vi "PosStrikerFollowAttacker.vi"(4 "Pos Attacker":dbl[](array[numeric]), 6 "atacando ao contrário?":bool=TRUE, 8 "IA Input":T1={"our_robots"=[], "enemy_robots"=[], "balls"=[], "geometry"={"line_width"=0, "field_length"=0, "field_width"=0, "boundary_width"=0, "referee_width"=0, "goal_width"=0, "goal_depth"=0, "goal_wall_width"=0, "center_circle_radius"=0, "defense_radius"=0, "defense_stretch"=0, "free_kick_from_defense_dist"=0, "penalty_spot_from_field_line_dist"=0, "penalty_line_from_spot_dist"=0}, "IA Judge"={"stage"="", "command"="", "our_goalie_id"=0.0, "enemy_goalie_id"=0.0, "command enum"=enum."Halt", "Time"=enum."Azul"}, "Received Timestamp"=timestamp(0 s since 1904-01-01), "Events"={"Touch"=FALSE, "Ball out"=FALSE, "id touch"=0.0, "Ball out of \nVision"=FALSE, "Ball inside \nGoalie area"=FALSE, "Robot not responding"=FALSE, "Robots responding status"=[1.0, 1.0, 1.0, 1.0, 1.0, 1.0], "Enemy Ball \nPossession"=FALSE, "Pass State"=FALSE, "id end of pass"=0.0, "Kick"=FALSE}}, 9 "balls":T5[](array[typedef])=[{"x"=-2165.869384765625, "y"=510.4085693359375, "timestamp"=timestamp(2082758857.4639893 s since 1904-01-01), "Vel_x"=0.0, "Vel_y"=0.0}], 10 "Field Size in":T6={"line_width"=10, "field_length"=6000, "field_width"=4000, "boundary_width"=250, "referee_width"=425, "goal_width"=700, "goal_depth"=180, "goal_wall_width"=20, "center_circle_radius"=500, "defense_radius"=500, "defense_stretch"=350, "free_kick_from_defense_dist"=700, "penalty_spot_from_field_line_dist"=450, "penalty_line_from_spot_dist"=350}, 11 "Robot in":T2={"id"=5, "function"=enum."Attacker", "x"=-1842.5054931640625, "y"=520.60986328125, "orientation"=-2.7555055618286133, "v_tangent"=0.0, "v_normal"=0.0, "v_ang"=0.0, "kick_x"=0.0, "kick_z"=0.0, "dribble"=FALSE, "Timestamp"=timestamp(2082758857.4639893 s since 1904-01-01), "dest_x"=0.0, "dest_y"=0.0, "dest_orientation"=0.0, "estimatives"={"est_v_tangent"=0.0, "est_v_normal"=0.0, "est_vx"=0.0, "est_vy"=0.0}, "dest_x_kick"=0.0, "dest_y_kick"=0.0, "Gap Coord"=[], "States"=enum."GoToTangent"}) -> (2 "Robot out":T2={"id"=5, "function"=enum."Attacker", "x"=-1842.5054931640625, "y"=520.60986328125, "orientation"=-2.7555055618286133, "v_tangent"=-0.08361641967936218, "v_normal"=-0.20513016702014014, "v_ang"=0.24456003022714357, "kick_x"=0.0, "kick_z"=0.0, "dribble"=FALSE, "Timestamp"=timestamp(2082758857.4639893 s since 1904-01-01), "dest_x"=0.0, "dest_y"=0.0, "dest_orientation"=0.0, "estimatives"={"est_v_tangent"=0.0, "est_v_normal"=0.0, "est_vx"=0.0, "est_vy"=0.0}, "dest_x_kick"=0.0, "dest_y_kick"=0.0, "Gap Coord"=[], "States"=enum."GoToTangent"})   [LabVIEW 2016]
uses:
  Core/AI Robot.ctl
  Functions Enum.ctl
  AttackerStates.ctl
  Core/Field Size.ctl
  Core/AI Ball.ctl
  Core/AI Input.ctl
  Core/AI Judge.ctl
  Command Enum.ctl
  Util/Events/Events.ctl
panel:
  in  "dist 2":dbl
  out "sentido":dbl
  in  "dist":dbl
  out "Yattacker":dbl
  out "Xattacker":dbl
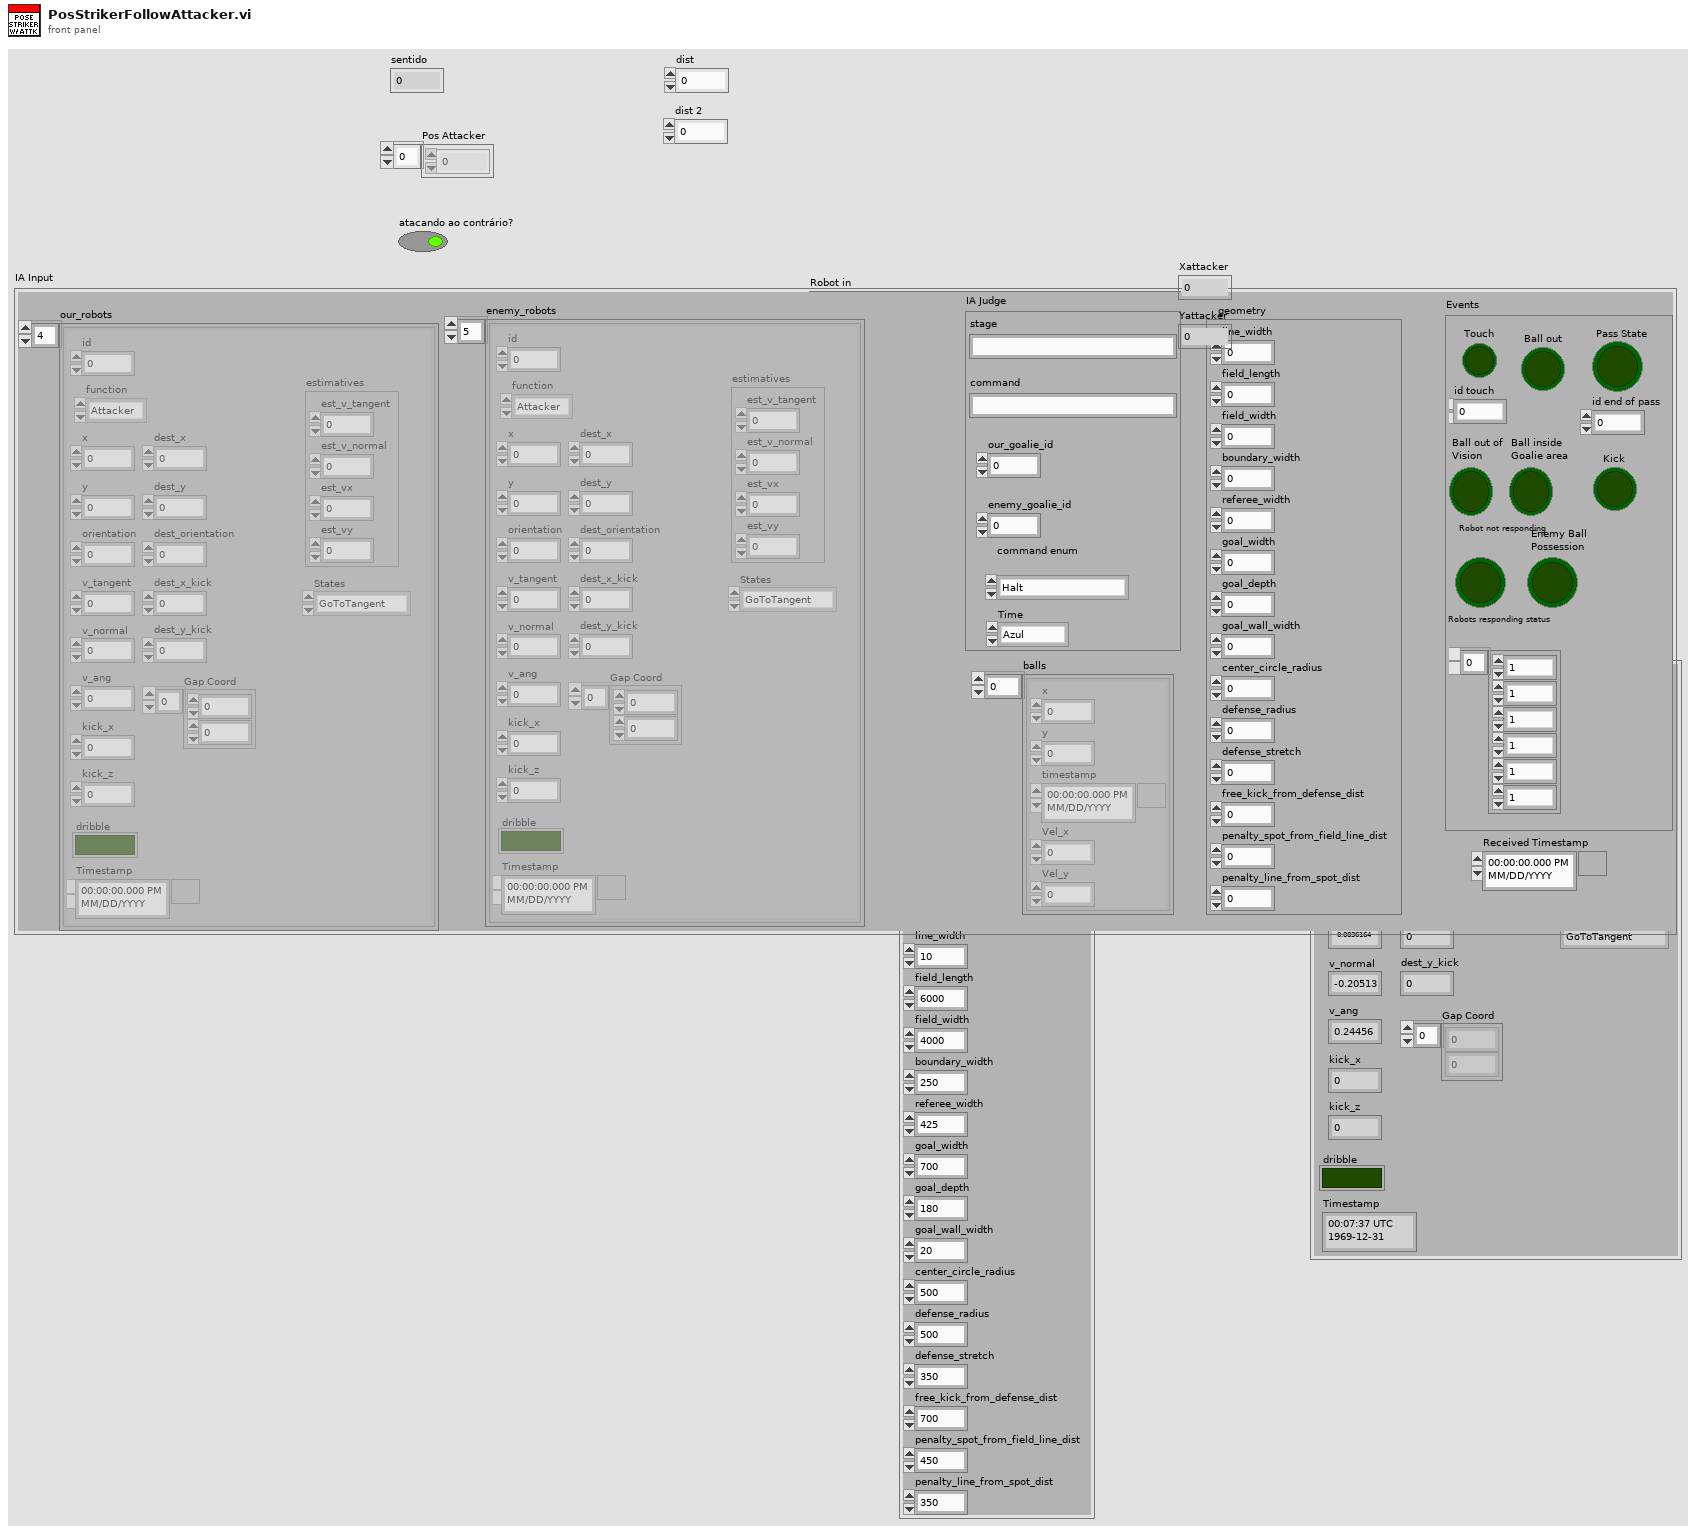
[diagram p1: front panel]
types:
  T1 = typedef "AI Input.ctl" = cluster{"our_robots":T2[], "enemy_robots":T2[], "balls":T5[], "geometry":T6, "IA Judge":T7, "Received Timestamp":timestamp, "Events":T9}
  T2 = typedef "AI Robot.ctl" = cluster{"id":u32, "function":T3, "x":dbl, "y":dbl, "orientation":dbl, "v_tangent":dbl, "v_normal":dbl, "v_ang":dbl, "kick_x":dbl, "kick_z":dbl, "dribble":bool, "Timestamp":timestamp, "dest_x":dbl, "dest_y":dbl, "dest_orientation":dbl, "estimatives":cluster{"est_v_tangent":dbl, "est_v_normal":dbl, "est_vx":dbl, "est_vy":dbl}, "dest_x_kick":dbl, "dest_y_kick":dbl, "Gap Coord":dbl[], "States":T4}
  T3 = typedef "Functions Enum.ctl" = enum16{"Attacker", "Goalie", "Defender", "Striker", "Goto 0", "Dummy", "Kicker", "ZigZag"}
  T4 = typedef "AttackerStates.ctl" = enum16{"Pass", "GoToTangent", "BallGetting", "GoToKick", ""}
  T5 = typedef "AI Ball.ctl" = cluster{"x":dbl, "y":dbl, "timestamp":timestamp, "Vel_x":dbl, "Vel_y":dbl}
  T6 = typedef "Field Size.ctl" = cluster{"line_width":u32, "field_length":u32, "field_width":u32, "boundary_width":u32, "referee_width":u32, "goal_width":u32, "goal_depth":u32, "goal_wall_width":u32, "center_circle_radius":u32, "defense_radius":u32, "defense_stretch":u32, "free_kick_from_defense_dist":u32, "penalty_spot_from_field_line_dist":u32, "penalty_line_from_spot_dist":u32}
  T7 = typedef "AI Judge.ctl" = cluster{"stage":string, "command":string, "our_goalie_id":dbl, "enemy_goalie_id":dbl, "command enum":T8, "Time":enum16{"Azul", "Amarelo"}}
  T8 = typedef "Command Enum.ctl" = enum16{"Halt", "Stop", "Force Start", "PKA Normal Start", "Prepare Kickoff Ally", "PKE Normal Start", "Prepare Kickoff Enemy", "Prepare Penalty Ally", "PPA Normal Start", "Prepare Penalty Enemy", "PPE Normal Start", "Direct Free Enemy", "Direct Free Ally", "Indirect Free Enemy", "Indirect Free Ally", "Timeout Enemy", "Timeout Ally", "Goal Enemy", "Goal Ally", "Ball Placement Enemy", "Ball Placement Ally", "Normal Half Time", "Extra Time Break", "Extra Half Time", "None"}
  T9 = typedef "Events.ctl" = cluster{"Touch":bool, "Ball out":bool, "id touch":dbl, "Ball out of \nVision":bool, "Ball inside \nGoalie area":bool, "Robot not responding":bool, "Robots responding status":dbl[], "Enemy Ball \nPossession":bool, "Pass State":bool, "id end of pass":dbl, "Kick":bool}
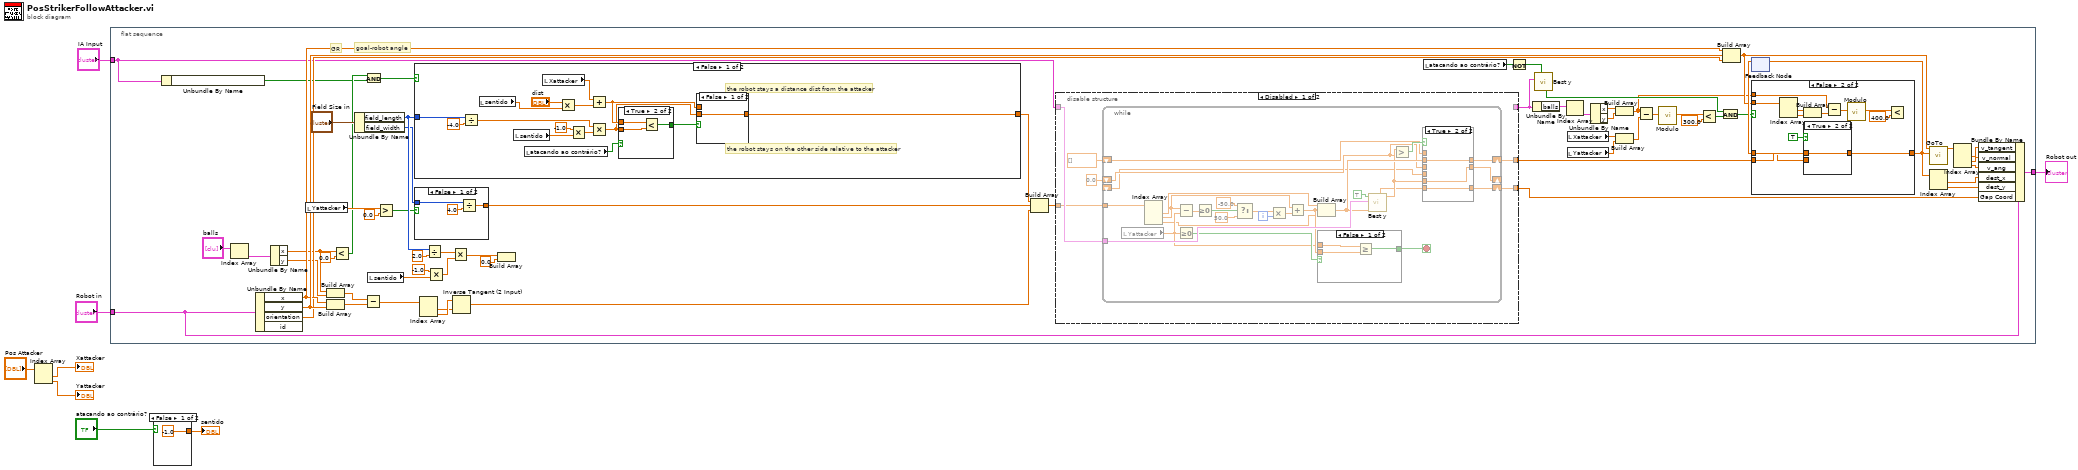
[diagram p0: block diagram]
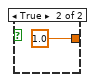
[diagram p2: hidden frame]
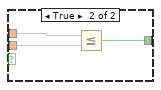
[diagram p5: hidden frame]
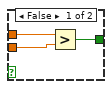
[diagram p8: hidden frame]
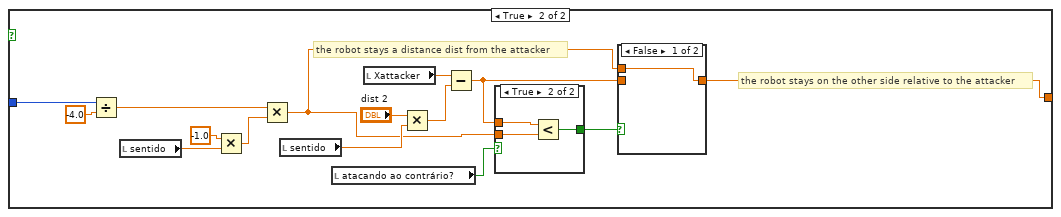
[diagram p10: hidden frame]
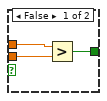
[diagram p11: hidden frame]
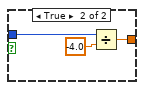
[diagram p13: hidden frame]
diagram:
  n1 = Index Array(array="Pos Attacker") -> (element #1=→"Xattacker":dbl, element #2=→"Yattacker":dbl)  [unwired: 2 in]
  n2 = flat-sequence {
    tunnel: [w52] -> w8
    tunnel: "Robot in" -> [w50]
    tunnel: "IA Input" -> [w9]
    frame #0 {
      # "GR"
      # "goal-robot angle"
      n3 = Unbundle By Name(w9) -> ("Events.Ball inside \nGoalie area"=w36:bool)
      n4 = Index Array(array="balls") -> (element=w40:T5)  [unwired: 1 in]
      n5 = Unbundle By Name(w50) -> ("x"=w66:dbl, "y"=w67:dbl, "orientation"=w53:dbl)  [unwired: 1 out]
      n6 = Unbundle By Name(w40) -> ("x"=w33:dbl, "y"=w32:dbl)
      n7 = local read "Yattacker"() -> (w51:dbl)
      n8 = Build Array(w33, w32) -> (w31:dbl[])
      n9 = Build Array(w66, w67) -> (w68:dbl[])
      n10 = Less?(x=w33, y=0.0) -> (x < y?=w37:bool)
      n11 = Unbundle By Name("Field Size in") -> ("field_length"=w70:u32, "field_width"=w57:u32)
      n12 = Subtract(x=w31, y=w68) -> (x-y=w65:dbl[])
      n13 = And(x=w37, y=w36) -> (x .and. y?=w38:bool)
      n14 = local read "sentido"() -> (w48:dbl)
      n15 = Greater?(x=w51, y=0.0) -> (0:w54:bool)
      n16 = case shown="False" w38 {
        tunnel: w70 -> [w149 w172]
        tunnel: [w148 w171] -> w59
        frame False {
          # "the robot stays on the other side relative to the attacker"
          # "the robot stays a distance dist from the attacker"
          n17 = Divide(x=w149, y=-4.0) -> (x/y=w146:dbl)
          n18 = local read "sentido"() -> (w139:dbl)
          n19 = local read "sentido"() -> (w142:dbl)
          n20 = local read "atacando ao contrário?"() -> (w138:bool)
          n21 = local read "Xattacker"() -> (w145:dbl)
          n22 = Multiply(x="dist", y=w139) -> (x*y=w144:dbl)
          n23 = Multiply(x=-1.0, y=w142) -> (x*y=w141:dbl)
          n24 = Add(x=w145, y=w144) -> (x+y=w137:dbl)
          n25 = Multiply(x=w146, y=w141) -> (x*y=w136:dbl)
          n26 = case shown="True" w138 {
            tunnel: w137 -> [w152 w154]
            tunnel: w136 -> [w151 w155]
            tunnel: [w150 w153] -> w135
            frame False {
              n27 = Greater?(x=w152, y=w151) -> (0:w150:bool)
            }
            frame True {
              n28 = Less?(x=w154, y=w155) -> (x < y?=w153:bool)
            }
          }
          n29 = case shown="False" w135 {
            tunnel: [w156 w157] -> w148
            tunnel: w137 -> [_ w157]
            tunnel: w136 -> [w156 _]
            frame False {
            }
            frame True {
            }
          }
        }
        frame True {
          # "the robot stays on the other side relative to the attacker"
          # "the robot stays a distance dist from the attacker"
          n30 = Divide(x=w172, y=-4.0) -> (x/y=w169:dbl)
          n31 = local read "sentido"() -> (w165:dbl)
          n32 = Multiply(x=-1.0, y=w165) -> (x*y=w164:dbl)
          n33 = Multiply(x=w169, y=w164) -> (x*y=w159:dbl)
          n34 = local read "sentido"() -> (w162:dbl)
          n35 = local read "atacando ao contrário?"() -> (w161:bool)
          n36 = local read "Xattacker"() -> (w168:dbl)
          n37 = Multiply(x="dist 2", y=w162) -> (x*y=w167:dbl)
          n38 = Subtract(x=w168, y=w167) -> (x-y=w160:dbl)
          n39 = case shown="True" w161 {
            tunnel: w160 -> [w175 w177]
            tunnel: w159 -> [w174 w178]
            tunnel: [w173 w176] -> w158
            frame False {
              n40 = Greater?(x=w175, y=w174) -> (0:w173:bool)
            }
            frame True {
              n41 = Less?(x=w177, y=w178) -> (x < y?=w176:bool)
            }
          }
          n42 = case shown="False" w158 {
            tunnel: [w179 w180] -> w171
            tunnel: w160 -> [_ w180]
            tunnel: w159 -> [w179 _]
            frame False {
            }
            frame True {
            }
          }
        }
      }
      n43 = case shown="False" w54 {
        tunnel: [w182 w185] -> w58
        tunnel: w57 -> [w181 w184]
        frame False {
          n44 = Divide(x=w181, y=4.0) -> (x/y=w182:dbl)
        }
        frame True {
          n45 = Divide(x=w184, y=-4.0) -> (x/y=w185:dbl)
        }
      }
      n46 = Index Array(array=w65) -> (element #1=w63:dbl, element #2=w64:dbl)  [unwired: 2 in]
      n47 = Divide(x=w70, y=2.0) -> (x/y=w46:dbl)
      n48 = Multiply(x=-1.0, y=w48) -> (x*y=w47:dbl)
      n49 = Multiply(x=w46, y=w47) -> (x*y=w45:dbl)
      n50 = Inverse Tangent (2 Input)(1:w63, 2:w64) -> (0:w72:dbl)
      n51 = Build Array(w45, 0.0 ("element")) -> ()  [unwired: 1 out]
      n52 = Build Array(w59, w58, w72) -> (w35:dbl[])
      n53 = disable-structure shown="Disabled" {
        disable-tunnel: w9 -> [w93 w133]
        disable-tunnel: w35 -> [w92 w134]
        disable-tunnel: [w91 w134] -> w30
        disable-tunnel: [w88 _] -> w34
        disable-tunnel: [_ w133] -> w25
        frame Disabled {
          n54 = while {
            tunnel: w93 -> [w115]
            shift-right: [w113] -> w91
            shift-left: dbl[] [] -> [w108]
            shift-right: [w111] -> _
            shift-left: 0.0 ("Gap kick") -> [w109]
            tunnel: w92 -> [w98]
            shift-right: [w97] -> w88
            shift-left: _ -> [w96]
            i -> [w118]
            stop <- w117 stop-if-true
            n55 = local read "Yattacker"() -> (w99:dbl)
            n56 = Index Array(array=w98) -> (element #1=w119:dbl, element #2=w107:dbl, element #3=w94:dbl)  [unwired: 3 in]
            n57 = Subtract(x=w107, y=w99) -> (x-y=w106:dbl)
            n58 = Greater Or Equal To 0?(x=w99) -> (x >= 0?=w100:bool)
            n59 = Greater Or Equal To 0?(x=w106) -> (x >= 0?=w105:bool)
            n60 = Select(t=-50.0, s=w105, f=50.0) -> (s? t:f=w102:dbl)
            n61 = Multiply(x=w102, y=w118) -> (x*y=w116:dbl)
            n62 = Add(x=w107, y=w116) -> (x+y=w101:dbl)
            n63 = Build Array(w119, w101, w94) -> (w114:dbl[])
            n64 = case shown="False" w100 {
              tunnel: [w123 w126] -> w117
              tunnel: w99 -> [w122 w125]
              tunnel: w101 -> [w121 w124]
              frame False {
                n65 = Greater Or Equal?(x=w122, y=w121) -> (x >= y?=w123:bool)
              }
              frame True {
                n66 = Less Or Equal?(x=w125, y=w124) -> (x <= y?=w126:bool)
              }
            }
            n67 = call "Best y.vi"("Ball false"=w114, "IA State"=w115, "Best y para varredura?"=TRUE) -> ("Gap kick"=w110:dbl, "Gap Coord"=w95:dbl[])  [unwired: 5 in, 2 out]
            n68 = Greater?(x=w110, y=w109) -> (0:w112:bool)
            n69 = case shown="True" w112 {
              tunnel: w114 -> [_ w132]
              tunnel: [w128 w132] -> w113
              tunnel: [w129 w131] -> w111
              tunnel: w110 -> [_ w131]
              tunnel: w109 -> [w129 _]
              tunnel: w108 -> [w128 _]
              tunnel: [w127 w130] -> w97
              tunnel: w96 -> [w127 _]
              tunnel: w95 -> [_ w130]
              frame False {
              }
              frame True {
              }
            }
          }
        }
        frame Enabled {
        }
      }
      n70 = local read "atacando ao contrário?"() -> (w26:bool)
      n71 = Not(x=w26) -> (.not. x?=w27:bool)
      n72 = Unbundle By Name(w25) -> ("balls"=w24:T5[])
      n73 = call "Best y.vi"("inimigos"=w27, "IA State"=w25) -> ("Eclipse"=w16:bool)  [unwired: 6 in, 3 out]
      n74 = Index Array(array=w24) -> (element=w23:T5)  [unwired: 1 in]
      n75 = local read "Xattacker"() -> (w20:dbl)
      n76 = local read "Yattacker"() -> (w19:dbl)
      n77 = Unbundle By Name(w23) -> ("x"=w22:dbl, "y"=w21:dbl)
      n78 = Build Array(w22, w21) -> (w10:dbl[])
      n79 = Build Array(w20, w19) -> (w18:dbl[])
      n80 = Subtract(x=w10, y=w18) -> (x-y=w17:dbl[])
      n81 = call "Modulo.vi"("2D vector"=w17) -> ("Modulo"=w13:dbl)  [unwired: 10 in]
      n82 = Less?(x=w13, y=300.0 ("x")) -> (x < y?=w14:bool)
      n83 = And(x=w16, y=w14) -> (x .and. y?=w15:bool)
      n84 = Build Array(w66, w67, w53) -> (w11:dbl[])
      n85 = feedback #1() -> (w28:dbl[])  [unwired: 1 in]
      n86 = case shown="False" w15 {
        tunnel: w30 -> [_ w76]
        tunnel: [w73 w77] -> w29
        tunnel: w28 -> [w73 w75]
        tunnel: w11 -> [_ w85]
        tunnel: w10 -> [_ w82]
        frame True {
        }
        frame False {
          n87 = Index Array(array=w85) -> (element #1=w84:dbl, element #2=w83:dbl)  [unwired: 2 in]
          n88 = Build Array(w84, w83) -> (w81:dbl[])
          n89 = case shown="True" TRUE {
            tunnel: [w86 w87] -> w77
            tunnel: w76 -> [_ w87]
            tunnel: w75 -> [w86 _]
            frame False {
            }
            frame True {
            }
          }
          n90 = Subtract(x=w82, y=w81) -> (x-y=w80:dbl[])
          n91 = call "Modulo.vi"("2D vector"=w80) -> ("Modulo"=w79:dbl)  [unwired: 10 in]
          n92 = Less?(x=w79, y=400.0) -> ()  [unwired: 1 out]
        }
      }
      n93 = feedback-in #1(w29) -> ()
      n94 = call "GoTo.vi"("Target"=w29, "Position"=w11) -> ("Output\nVelocity"=w44:dbl[])  [unwired: 8 in, 1 out]
      n95 = Index Array(array=w29) -> (element #1=w43:dbl, element #2=w42:dbl)  [unwired: 2 in]
      n96 = Index Array(array=w44) -> (element #1=w60:dbl, element #2=w62:dbl, element #3=w61:dbl)  [unwired: 3 in]
      n97 = Bundle By Name(cluster=w50, "v_tangent"=w60, "v_normal"=w62, "v_ang"=w61, "dest_x"=w43, "dest_y"=w42, "Gap Coord"=w34) -> (w52:T2)
    }
  }
  n98 = case shown="False" "atacando ao contrário?" {
    tunnel: [-1.0 1.0] -> w6
    frame False {
    }
    frame True {
    }
  }
  "sentido" <- w6
  "Robot out" <- w8
